vi "Get Bucket Location.vi"(8 "error in (no error)":errorcluster, 9 "Bucket":string) -> (0 "error out":errorcluster, 3 "Location":T1)   [LabVIEW 2011, in "LV Interface for Amazon S3.lvlib"]
doc: "This operation <B>returns</B> a <B>bucket's Region</B>. You set the bucket's Region using the LocationContraint request parameter in a PUT Bucket request. To use this implementation of the operation, <B>you must be the bucket Owner</B>."
uses:
  LV Interface for Amazon S3.lvlib
  Typedefs/AMZ_S3_LocationConstraint.ctl
  XML Parser/XML Parser.lvlib
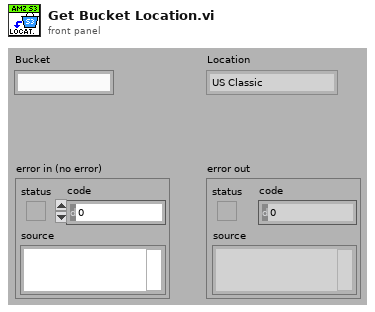
[diagram p1: front panel]
types:
  T1 = typedef "LV Interface for Amazon S3.lvlib/AMZ_S3_LocationConstraint.ctl" = enum16{"US Classic", "EU", "US-West-1", "AP-SouthEast-1"}
  T2 = typedef "LV Interface for Amazon S3.lvlib/AMZ_S3_Call Results.ctl" = enum16{"Success", "UndefinedError", "AccessDenied", "AccountProblem", "AmbiguousGrantByEmailAddress", "BadDigest", "BucketAlreadyExists", "BucketAlreadyOwnedByYou", "BucketNotEmpty", "CredentialsNotSupported", "CrossLocationLoggingProhibited", "EntityTooSmall", "EntityTooLarge", "ExpiredToken", "IllegalVersioningConfigurationException", "IncompleteBody", "IncorrectNumberOfFilesInPostRequest", "InlineDataTooLarge", "InternalError", "InvalidAccessKeyId", "InvalidAddressingHeader", "InvalidArgument", "InvalidBucketName", "InvalidDigest", "InvalidLocationConstraint", "InvalidPart", "InvalidPartOrder", "InvalidPayer", "InvalidPolicyDocument", "InvalidRange", "InvalidSecurity", "InvalidSOAPRequest", "InvalidStorageClass", "InvalidTargetBucketForLogging", "InvalidToken", "InvalidURI", "KeyTooLong", "MalformedACLError", "MalformedPOSTRequest", "MalformedXML", "MaxMessageLengthExceeded", "MaxPostPreDataLengthExceededError", "MetadataTooLarge", "MethodNotAllowed", "MissingAttachment", "MissingContentLength", "MissingRequestBodyError", "MissingSecurityElement", "MissingSecurityHeader", "NoLoggingStatusForKey", "NoSuchBucket", "NoSuchKey", "NoSuchUpload", "NoSuchVersion", "NotImplemented", "NotSignedUp", "OperationAborted", "PermanentRedirect", "PreconditionFailed", "Redirect", "RequestIsNotMultiPartContent", "RequestTimeout", "RequestTimeTooSkewed", "RequestTorrentOfBucketError", "SignatureDoesNotMatch", "SlowDown", "TemporaryRedirect", "TokenRefreshRequired", "TooManyBuckets", "UnexpectedContent", "UnresolvableGrantByEmailAddress", "UserKeyMustBeSpecified", "LabVIEWError"}
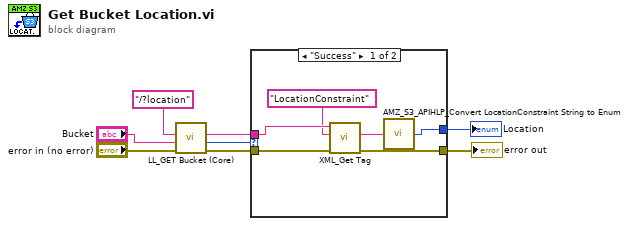
[diagram p0: block diagram]
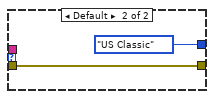
[diagram p2: hidden frame]
diagram:
  n1 = call "LL_GET Bucket (Core).vi"("error in (no error)"="error in (no error)", "Bucket"="Bucket", "Path and query string"="/?location") -> ("error out"=w4:errorcluster, "Call Result"=w5:T2, "Response body"=w3:string)  [unwired: 5 in, 1 out]
  n2 = case shown="\"Success\"" w5 {
    tunnel: w4 -> [w14 w16]
    tunnel: w3 -> [w13 _]
    tunnel: [w11 w16] -> w2
    tunnel: [w9 AMZ_S3_LocationConstraint."US Classic" ("Location")] -> w1
    frame "Success" {
      n3 = call "XML_Get Tag.vi"("error in (no error)"=w14, "Tag name"="LocationConstraint", "XML String in"=w13) -> ("error out"=w11:errorcluster, "Tag value"=w10:string)  [unwired: 4 in, 3 out]
      n4 = call "AMZ_S3_APIHLP_Convert LocationConstraint String to Enum.vi"("Location String"=w10) -> ("Location"=w9:T1)  [unwired: 4 in]
    }
    frame Default {
    }
  }
  "error out" <- w2
  "Location" <- w1
